vi "Check Start Move.vi"(0 "Bd ID In":T6, 1 "Start All (False)":bool, 2 "Run Mode":enum32{"Sequential", "Parallel"}(ring), 5 "Axis Controls":T1={"Axis 1"={"Axis"=1, "Enable"=FALSE, "Start"=FALSE, "Home"=FALSE, "Stop Type"=0, "Kill"=FALSE}, "Axis 2"={"Axis"=1, "Enable"=FALSE, "Start"=FALSE, "Home"=FALSE, "Stop Type"=0, "Kill"=FALSE}, "Axis 3"={"Axis"=1, "Enable"=FALSE, "Start"=FALSE, "Home"=FALSE, "Stop Type"=0, "Kill"=FALSE}, "Axis 4"={"Axis"=1, "Enable"=FALSE, "Start"=FALSE, "Home"=FALSE, "Stop Type"=0, "Kill"=FALSE}, "Axis 5"={"Axis"=1, "Enable"=FALSE, "Start"=FALSE, "Home"=FALSE, "Stop Type"=0, "Kill"=FALSE}, "Axis 6"={"Axis"=1, "Enable"=FALSE, "Start"=FALSE, "Home"=FALSE, "Stop Type"=0, "Kill"=FALSE}} {"Axis 6"."Stop Type" items=["Decelerate", "Halt", "Kill"]; "Axis 6"."Axis" items=["Axis 1"=1, "Axis 2"=2, "Axis 3"=3, "Axis 4"=4, "Axis 5"=5, "Axis 6"=6, "Axis 7"=7, "Axis 8"=8]; "Axis 5"."Stop Type" items=["Decelerate", "Halt", "Kill"]; "Axis 5"."Axis" items=["Axis 1"=1, "Axis 2"=2, "Axis 3"=3, "Axis 4"=4, "Axis 5"=5, "Axis 6"=6, "Axis 7"=7, "Axis 8"=8]; "Axis 4"."Stop Type" items=["Decelerate", "Halt", "Kill"]; "Axis 4"."Axis" items=["Axis 1"=1, "Axis 2"=2, "Axis 3"=3, "Axis 4"=4, "Axis 5"=5, "Axis 6"=6, "Axis 7"=7, "Axis 8"=8]; "Axis 3"."Stop Type" items=["Decelerate", "Halt", "Kill"]; "Axis 3"."Axis" items=["Axis 1"=1, "Axis 2"=2, "Axis 3"=3, "Axis 4"=4, "Axis 5"=5, "Axis 6"=6, "Axis 7"=7, "Axis 8"=8]; "Axis 2"."Stop Type" items=["Decelerate", "Halt", "Kill"]; "Axis 2"."Axis" items=["Axis 1"=1, "Axis 2"=2, "Axis 3"=3, "Axis 4"=4, "Axis 5"=5, "Axis 6"=6, "Axis 7"=7, "Axis 8"=8]; "Axis 1"."Stop Type" items=["Decelerate", "Halt", "Kill"]; "Axis 1"."Axis" items=["Axis 1"=1, "Axis 2"=2, "Axis 3"=3, "Axis 4"=4, "Axis 5"=5, "Axis 6"=6, "Axis 7"=7, "Axis 8"=8]}, 7 "Units (Encoder Counts)":T5=enum."Degrees", 9 "Stop refnum array":refnum<vi>[](array[refnum]), 11 "error in":errorcluster, 12 "Trajectory Parameters":T4={"Operation Mode (Absolute)"=0, "Blend"=FALSE, "Velocity"=6.0, "Acceleration"=4.0, "Deceleration"=4.0, "Blend Factor"=0, "Permitted Following Error"=1000.0, "S Curve Time"=0} {"Operation Mode (Absolute)" items=["Absolute Position", "Relative Position"]}, 13 "Target Positions":dbl[][](array[numeric])) -> (4 "Bd ID Out":T6, 15 "error out":errorcluster)   [LabVIEW 2010]
doc: "Written specifically for the MultiAxisMove VI. Polls the 'Controls' cluster for a 'Start' or 'Start All' signal. If 'Start All' is true, the singleAxisMultiMove subVI is called for all axes in parallel or sequentially depending on the Run Mode parameter. Otherwise, function checks for a true 'Start' condition on each axes in parallel and calls the singleAxisMultiMove subVI accordingly. \n\nTarget Position is a 2D array where each column is an array of positions for the corresponding axis. That is, the first column is an array of positions for the first axis, the second column is an array of positions for the second axis, etc. etc."
uses:
  Typedefs/Units_Enum.ctl
  Shared/typedefs/Trajectory Parameters.ctl
  Typedefs/AxisSpaceControls_ClusterofAxisControls.ctl
  Typedefs/AxisControls_cluster.ctl
  <vilib>/Motion/FlexMotion/CustomControls/CustomControls.llb/Axis To Control.flx
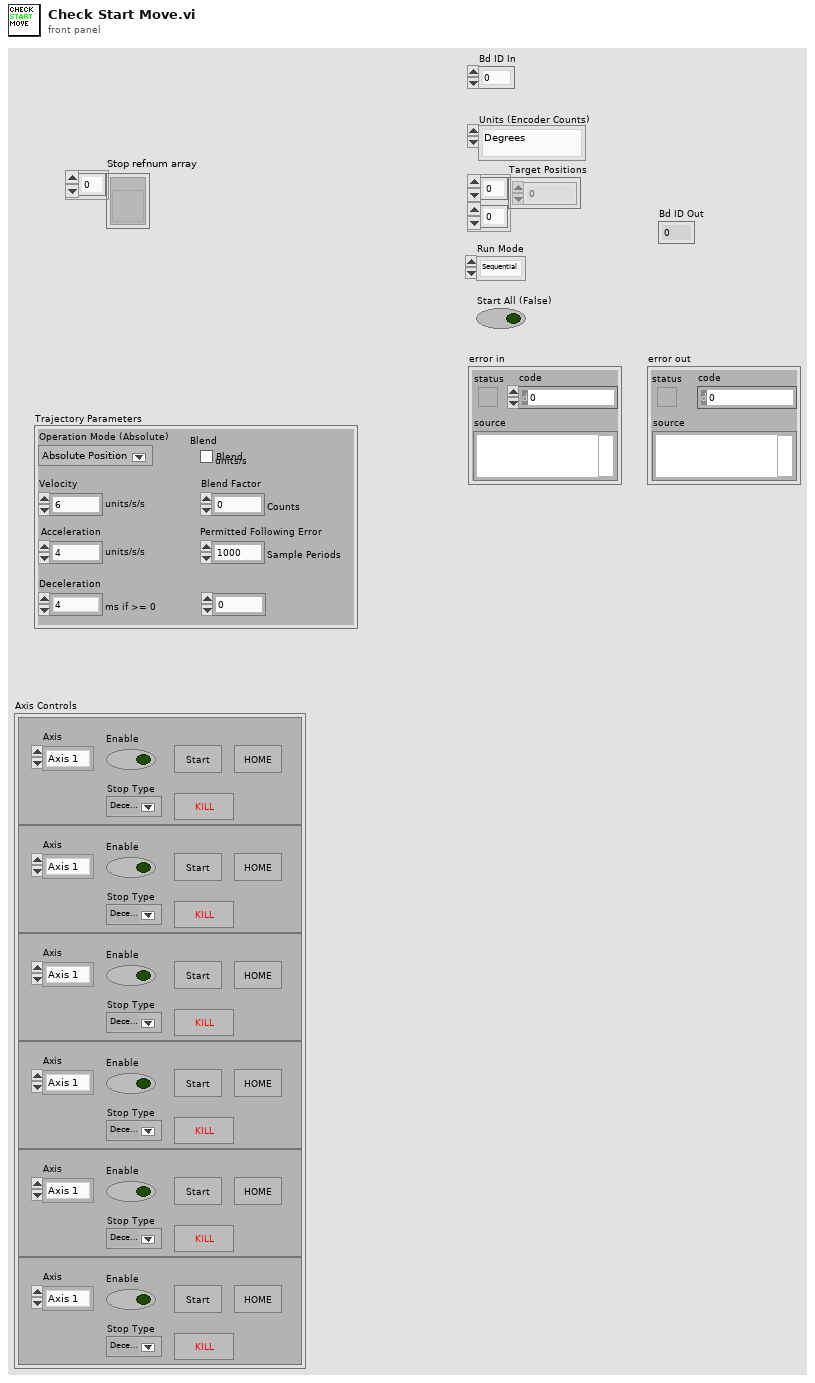
[diagram p1: front panel]
types:
  T1 = typedef "AxisSpaceControls_ClusterofAxisControls.ctl" = cluster{"Axis 1":T2, "Axis 2":T2, "Axis 3":T2, "Axis 4":T2, "Axis 5":T2, "Axis 6":T2}
  T2 = typedef "AxisControls_cluster.ctl" = cluster{"Axis":T3, "Enable":bool, "Start":bool, "Home":bool, "Stop Type":u16, "Kill":bool}
  T3 = typedef "Axis To Control.flx" = u16
  T4 = typedef "Trajectory Parameters.ctl" = cluster{"Operation Mode (Absolute)":u16, "Blend":bool, "Velocity":dbl, "Acceleration":dbl, "Deceleration":dbl, "Blend Factor":i16, "Permitted Following Error":dbl, "S Curve Time":u16}
  T5 = typedef "Units_Enum.ctl" = enum16{"Radians", "Encoder Counts", "Revolutions", "Degrees"}
  T6 = typedef "Bd Id Out" = u8
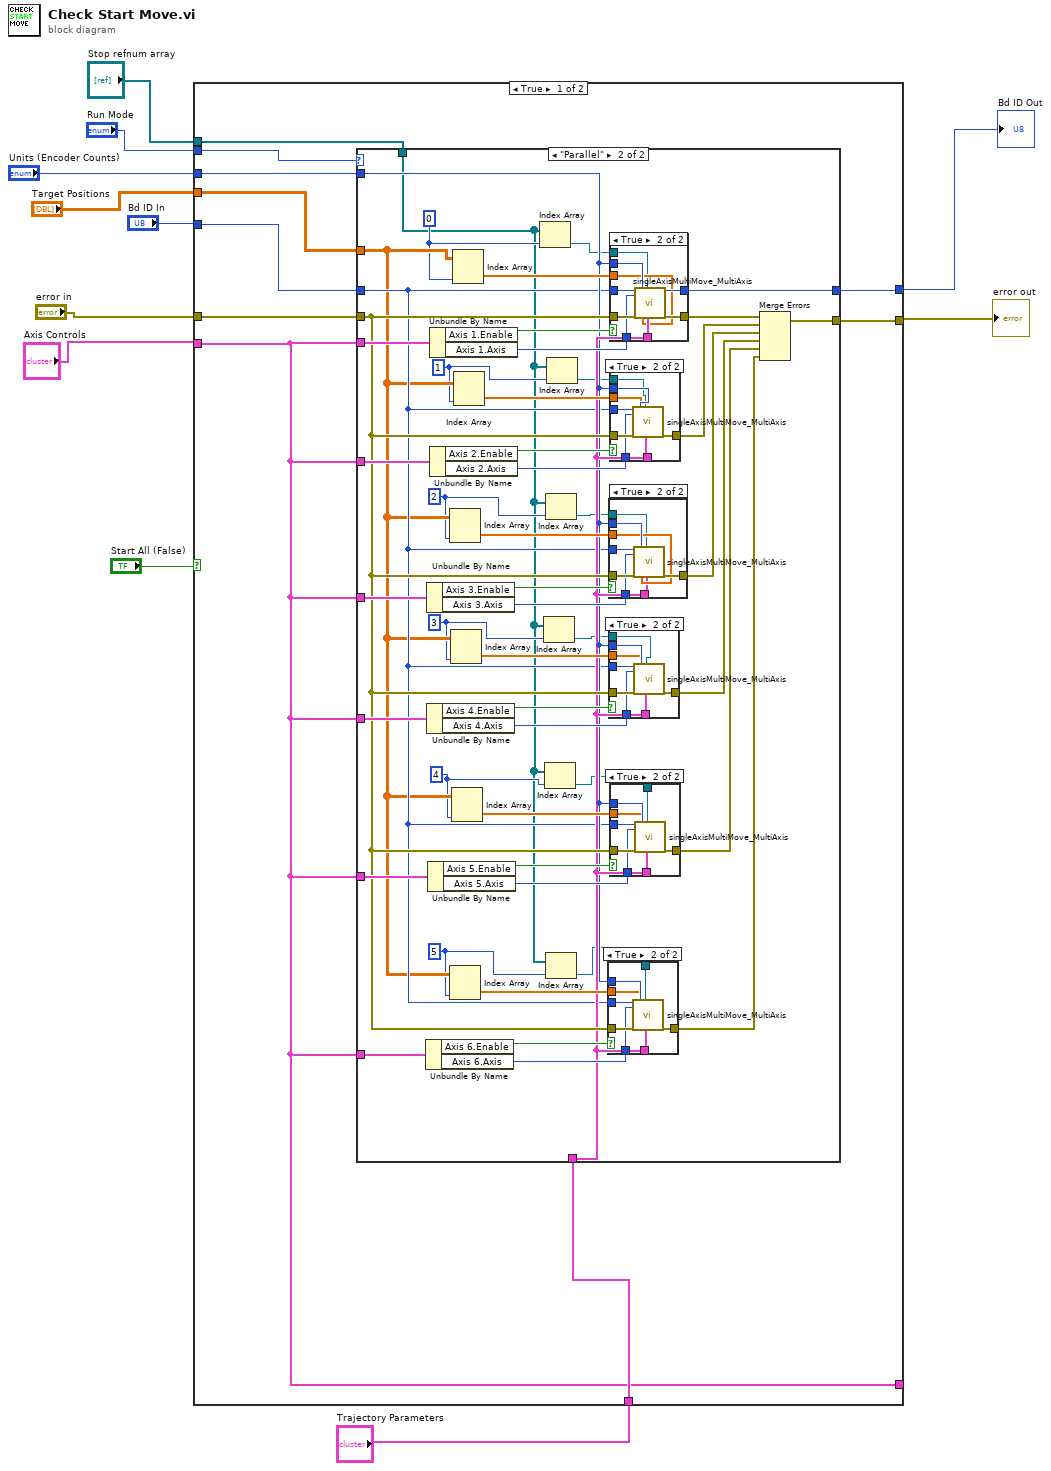
[diagram p0: block diagram]
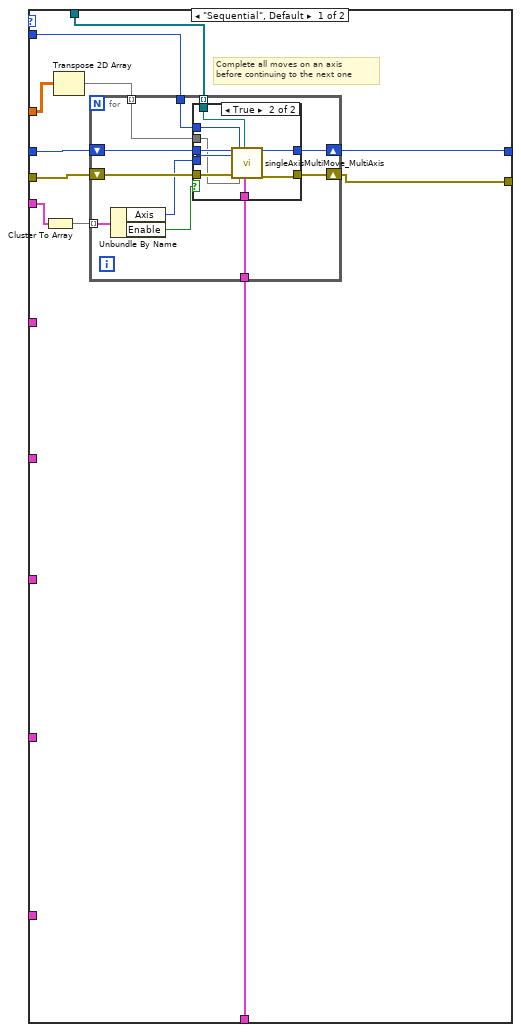
[diagram p2: hidden frame]
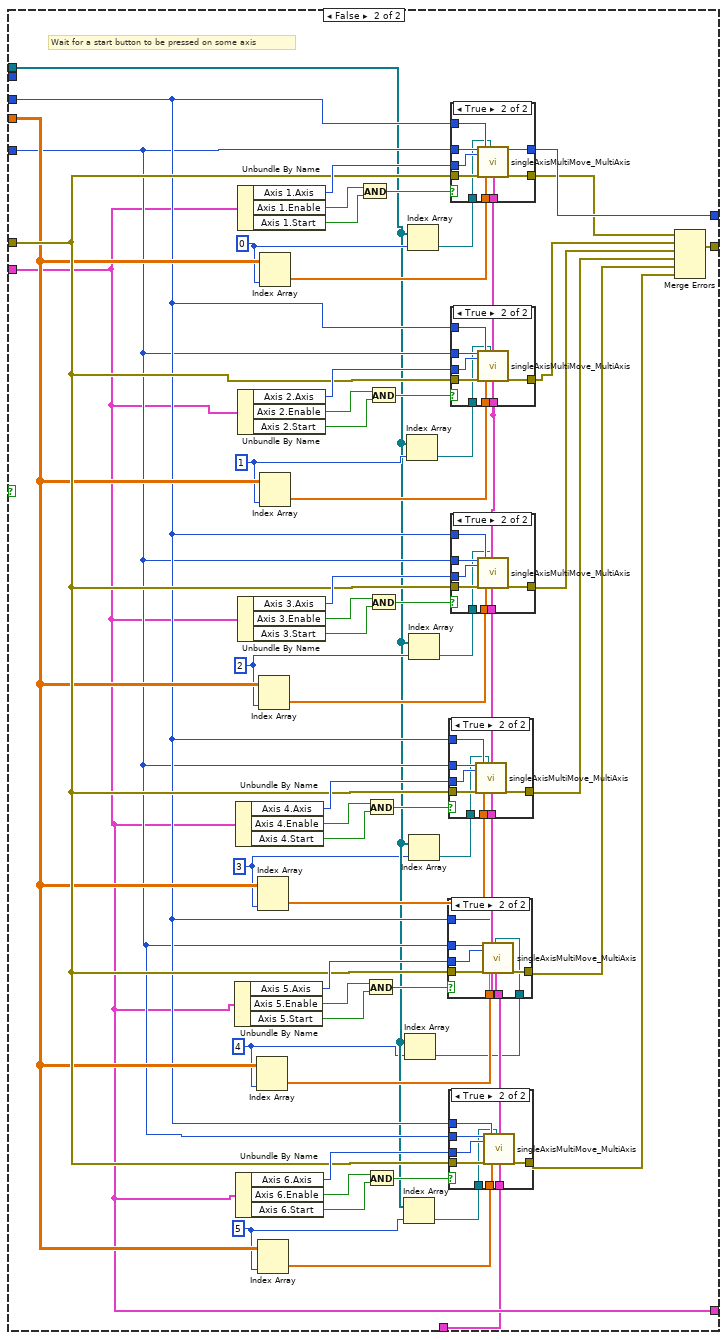
[diagram p10: hidden frame]
diagram:
  n1 = case shown="True" "Start All (False)" {
    tunnel: "Bd ID In" -> [w15 w177]
    tunnel: "error in" -> [w20 w180]
    tunnel: "Target Positions" -> [w17 w179]
    tunnel: "Run Mode" -> [w21 _]
    tunnel: "Axis Controls" -> [w16 w176]
    tunnel: "Trajectory Parameters" -> [w19 w174]
    tunnel: [w18 w216] -> w9
    tunnel: [w16 w176] -> _
    tunnel: [w14 w217] -> w6
    tunnel: "Units (Encoder Counts)" -> [w13 w178]
    tunnel: "Stop refnum array" -> [w12 w167]
    frame True {
      n2 = case shown="\"Parallel\"" w21 {
        tunnel: w20 -> [w32 w73]
        tunnel: w17 -> [w31 w68]
        tunnel: w16 -> [w29 w104]
        tunnel: w15 -> [w28 w70]
        tunnel: w19 -> [w26 w72]
        tunnel: [w25 w102] -> w18
        tunnel: w16 -> [_ w97]
        tunnel: w16 -> [_ w87]
        tunnel: w16 -> [_ w86]
        tunnel: w16 -> [_ w79]
        tunnel: w16 -> [_ w74]
        tunnel: [w24 w83] -> w14
        tunnel: w13 -> [w23 w71]
        tunnel: w12 -> [w22 w56]
        frame "Sequential", Default {
          # "Complete all moves on an axis\nbefore continuing to the next one"
          n3 = Cluster To Array(cluster=w29) -> (array=w27:T2[])
          n4 = Transpose 2D Array(2D array=w31) -> (transposed array=w30:dbl[][])
          n5 = for {
            tunnel: w30 -> [w37] mode=indexing
            tunnel: w27 -> [w41] mode=indexing
            tunnel: w26 -> [w38]
            shift-right: [w36] -> w25
            shift-left: w32 -> [w43]
            tunnel: w23 -> [w35]
            shift-right: [w34] -> w24
            shift-left: w28 -> [w42]
            tunnel: w22 -> [w33] mode=indexing
            n6 = Unbundle By Name(w41) -> ("Axis"=w40:T3, "Enable"=w39:bool)
            n7 = case shown="True" w39 {
              tunnel: w43 -> [w45 w54]
              tunnel: w42 -> [w44 w53]
              tunnel: w40 -> [_ w52]
              tunnel: w38 -> [_ w48]
              tunnel: w37 -> [_ w47]
              tunnel: [w45 w51] -> w36
              tunnel: w35 -> [_ w49]
              tunnel: [w44 w50] -> w34
              tunnel: w33 -> [_ w46]
              frame False {
              }
              frame True {
                n8 = call "singleAxisMultiMove_MultiAxis.vi"("Bd ID"=w53, "Axis"=w52, "error in (no error)"=w54, "Units (Encoder Counts)"=w49, "Target Positions"=w47, "Stop Refnum"=w46, "Trajectory Parameters"=w48) -> ("Bd ID Out"=w50:T6, "error out"=w51:errorcluster)  [unwired: 10 in, 1 out]
              }
            }
          }
        }
        frame "Parallel" {
          w57 = 5 ("disabled index (col)")
          w59 = 4 ("disabled index (col)")
          w61 = 3 ("disabled index (col)")
          w63 = 2 ("disabled index (col)")
          w65 = 1 ("disabled index (col)")
          w66 = 0 ("disabled index (col)")
          n9 = Unbundle By Name(w74) -> ("Axis 6.Enable"=w77:bool, "Axis 6.Axis"=w76:T3)
          n10 = Unbundle By Name(w87) -> ("Axis 3.Enable"=w89:bool, "Axis 3.Axis"=w88:T3)
          n11 = Unbundle By Name(w86) -> ("Axis 4.Enable"=w90:bool, "Axis 4.Axis"=w91:T3)
          n12 = Unbundle By Name(w79) -> ("Axis 5.Enable"=w80:bool, "Axis 5.Axis"=w81:T3)
          n13 = Unbundle By Name(w104) -> ("Axis 1.Enable"=w95:bool, "Axis 1.Axis"=w94:T3)
          n14 = Unbundle By Name(w97) -> ("Axis 2.Enable"=w96:bool, "Axis 2.Axis"=w98:T3)
          n15 = Index Array(array=w68, index (col)=w63) -> (element=w93:dbl[])  [unwired: 1 in]
          n16 = Index Array(array=w68, index (col)=w57) -> (element=w75:dbl[])  [unwired: 1 in]
          n17 = Index Array(array=w68, index (col)=w61) -> (element=w92:dbl[])  [unwired: 1 in]
          n18 = Index Array(array=w68, index (col)=w59) -> (element=w82:dbl[])  [unwired: 1 in]
          n19 = Index Array(array=w68, index (col)=w66) -> (element=w103:dbl[])  [unwired: 1 in]
          n20 = Index Array(array=w68, index (col)=w65) -> (element=w99:dbl[])  [unwired: 1 in]
          n21 = Index Array(array=w56, index=w66) -> (element=w67:refnum<vi>)
          n22 = Index Array(array=w56, index=w61) -> (element=w60:refnum<vi>)
          n23 = Index Array(array=w56, index=w59) -> (element=w58:refnum<vi>)
          n24 = Index Array(array=w56, index=w63) -> (element=w62:refnum<vi>)
          n25 = Index Array(array=w56, index=w57) -> (element=w55:refnum<vi>)
          n26 = Index Array(array=w56, index=w65) -> (element=w64:refnum<vi>)
          n27 = case shown="True" w77 {
            tunnel: w73 -> [w105 w113]
            tunnel: w72 -> [_ w108]
            tunnel: [w105 w112] -> w69
            tunnel: w70 -> [_ w111]
            tunnel: w75 -> [_ w107]
            tunnel: w76 -> [_ w110]
            tunnel: w71 -> [_ w109]
            tunnel: w55 -> [_ w106]
            frame False {
            }
            frame True {
              n28 = call "singleAxisMultiMove_MultiAxis.vi"("Bd ID"=w111, "Axis"=w110, "error in (no error)"=w113, "Units (Encoder Counts)"=w109, "Target Positions"=w107, "Stop Refnum"=w106, "Trajectory Parameters"=w108) -> ("error out"=w112:errorcluster)  [unwired: 10 in, 2 out]
            }
          }
          n29 = case shown="True" w89 {
            tunnel: w73 -> [w132 w140]
            tunnel: w70 -> [_ w139]
            tunnel: w93 -> [_ w135]
            tunnel: w72 -> [_ w134]
            tunnel: [w132 w138] -> w85
            tunnel: w88 -> [_ w137]
            tunnel: w71 -> [_ w136]
            tunnel: w62 -> [_ w133]
            frame False {
            }
            frame True {
              n30 = call "singleAxisMultiMove_MultiAxis.vi"("Bd ID"=w139, "Axis"=w137, "error in (no error)"=w140, "Units (Encoder Counts)"=w136, "Target Positions"=w135, "Stop Refnum"=w133, "Trajectory Parameters"=w134) -> ("error out"=w138:errorcluster)  [unwired: 10 in, 2 out]
            }
          }
          n31 = case shown="True" w90 {
            tunnel: w73 -> [w123 w131]
            tunnel: w72 -> [_ w126]
            tunnel: [w123 w130] -> w84
            tunnel: w70 -> [_ w129]
            tunnel: w92 -> [_ w125]
            tunnel: w91 -> [_ w128]
            tunnel: w71 -> [_ w127]
            tunnel: w60 -> [_ w124]
            frame False {
            }
            frame True {
              n32 = call "singleAxisMultiMove_MultiAxis.vi"("Bd ID"=w129, "Axis"=w128, "error in (no error)"=w131, "Units (Encoder Counts)"=w127, "Target Positions"=w125, "Stop Refnum"=w124, "Trajectory Parameters"=w126) -> ("error out"=w130:errorcluster)  [unwired: 10 in, 2 out]
            }
          }
          n33 = case shown="True" w95 {
            tunnel: w73 -> [w151 w160]
            tunnel: w70 -> [w150 w159]
            tunnel: w103 -> [_ w153]
            tunnel: w72 -> [_ w154]
            tunnel: [w151 w158] -> w100
            tunnel: w94 -> [_ w157]
            tunnel: w71 -> [_ w155]
            tunnel: [w150 w156] -> w83
            tunnel: w67 -> [_ w152]
            frame False {
            }
            frame True {
              n34 = call "singleAxisMultiMove_MultiAxis.vi"("Bd ID"=w159, "Axis"=w157, "error in (no error)"=w160, "Units (Encoder Counts)"=w155, "Target Positions"=w153, "Stop Refnum"=w152, "Trajectory Parameters"=w154) -> ("Bd ID Out"=w156:T6, "error out"=w158:errorcluster)  [unwired: 10 in, 1 out]
            }
          }
          n35 = case shown="True" w96 {
            tunnel: w73 -> [w141 w149]
            tunnel: w72 -> [_ w144]
            tunnel: [w141 w148] -> w101
            tunnel: w70 -> [_ w147]
            tunnel: w99 -> [_ w143]
            tunnel: w98 -> [_ w146]
            tunnel: w71 -> [_ w145]
            tunnel: w64 -> [_ w142]
            frame False {
            }
            frame True {
              n36 = call "singleAxisMultiMove_MultiAxis.vi"("Bd ID"=w147, "Axis"=w146, "error in (no error)"=w149, "Units (Encoder Counts)"=w145, "Target Positions"=w143, "Stop Refnum"=w142, "Trajectory Parameters"=w144) -> ("error out"=w148:errorcluster)  [unwired: 10 in, 2 out]
            }
          }
          n37 = case shown="True" w80 {
            tunnel: w73 -> [w114 w122]
            tunnel: w72 -> [_ w117]
            tunnel: [w114 w121] -> w78
            tunnel: w70 -> [_ w120]
            tunnel: w82 -> [_ w116]
            tunnel: w81 -> [_ w119]
            tunnel: w71 -> [_ w118]
            tunnel: w58 -> [_ w115]
            frame False {
            }
            frame True {
              n38 = call "singleAxisMultiMove_MultiAxis.vi"("Bd ID"=w120, "Axis"=w119, "error in (no error)"=w122, "Units (Encoder Counts)"=w118, "Target Positions"=w116, "Stop Refnum"=w115, "Trajectory Parameters"=w117) -> ("error out"=w121:errorcluster)  [unwired: 10 in, 2 out]
            }
          }
          n39 = Merge Errors(w100, w101, w85, w84, w78, w69) -> (w102:errorcluster)
        }
      }
    }
    frame False {
      w166 = 5 ("disabled index (col)")
      w163 = 4 ("disabled index (col)")
      w162 = 3 ("disabled index (col)")
      w169 = 2 ("disabled index (col)")
      w171 = 1 ("disabled index (col)")
      w172 = 0 ("disabled index (col)")
      # "Wait for a start button to be pressed on some axis"
      n40 = Unbundle By Name(w176) -> ("Axis 5.Axis"=w189:T3, "Axis 5.Enable"=w190:bool, "Axis 5.Start"=w187:bool)
      n41 = Unbundle By Name(w176) -> ("Axis 4.Axis"=w194:T3, "Axis 4.Enable"=w195:bool, "Axis 4.Start"=w192:bool)
      n42 = Unbundle By Name(w176) -> ("Axis 6.Axis"=w184:T3, "Axis 6.Enable"=w185:bool, "Axis 6.Start"=w182:bool)
      n43 = Unbundle By Name(w176) -> ("Axis 1.Axis"=w209:T3, "Axis 1.Enable"=w210:bool, "Axis 1.Start"=w207:bool)
      n44 = Unbundle By Name(w176) -> ("Axis 2.Axis"=w204:T3, "Axis 2.Enable"=w205:bool, "Axis 2.Start"=w202:bool)
      n45 = Unbundle By Name(w176) -> ("Axis 3.Axis"=w199:T3, "Axis 3.Enable"=w200:bool, "Axis 3.Start"=w197:bool)
      n46 = Index Array(array=w179, index (col)=w163) -> (element=w188:dbl[])  [unwired: 1 in]
      n47 = Index Array(array=w179, index (col)=w162) -> (element=w193:dbl[])  [unwired: 1 in]
      n48 = Index Array(array=w179, index (col)=w166) -> (element=w183:dbl[])  [unwired: 1 in]
      n49 = Index Array(array=w179, index (col)=w169) -> (element=w198:dbl[])  [unwired: 1 in]
      n50 = Index Array(array=w179, index (col)=w172) -> (element=w208:dbl[])  [unwired: 1 in]
      n51 = Index Array(array=w179, index (col)=w171) -> (element=w203:dbl[])  [unwired: 1 in]
      n52 = And(x=w210, y=w207) -> (x .and. y?=w211:bool)
      n53 = And(x=w190, y=w187) -> (x .and. y?=w191:bool)
      n54 = And(x=w195, y=w192) -> (x .and. y?=w196:bool)
      n55 = And(x=w185, y=w182) -> (x .and. y?=w186:bool)
      n56 = And(x=w205, y=w202) -> (x .and. y?=w206:bool)
      n57 = And(x=w200, y=w197) -> (x .and. y?=w201:bool)
      n58 = Index Array(array=w167, index=w166) -> (element=w165:refnum<vi>)
      n59 = Index Array(array=w167, index=w163) -> (element=w164:refnum<vi>)
      n60 = Index Array(array=w167, index=w171) -> (element=w170:refnum<vi>)
      n61 = Index Array(array=w167, index=w172) -> (element=w173:refnum<vi>)
      n62 = Index Array(array=w167, index=w169) -> (element=w168:refnum<vi>)
      n63 = Index Array(array=w167, index=w162) -> (element=w161:refnum<vi>)
      n64 = case shown="True" w191 {
        tunnel: w177 -> [_ w235]
        tunnel: [w227 w234] -> w181
        tunnel: w180 -> [w227 w233]
        tunnel: w178 -> [_ w229]
        tunnel: w189 -> [_ w232]
        tunnel: w188 -> [_ w230]
        tunnel: w174 -> [_ w231]
        tunnel: w164 -> [_ w228]
        frame False {
        }
        frame True {
          n65 = call "singleAxisMultiMove_MultiAxis.vi"("Bd ID"=w235, "Axis"=w232, "error in (no error)"=w233, "Units (Encoder Counts)"=w229, "Target Positions"=w230, "Stop Refnum"=w228, "Trajectory Parameters"=w231) -> ("error out"=w234:errorcluster)  [unwired: 10 in, 2 out]
        }
      }
      n66 = case shown="True" w196 {
        tunnel: w177 -> [_ w244]
        tunnel: [w236 w243] -> w212
        tunnel: w180 -> [w236 w242]
        tunnel: w178 -> [_ w240]
        tunnel: w194 -> [_ w241]
        tunnel: w193 -> [_ w239]
        tunnel: w174 -> [_ w238]
        tunnel: w161 -> [_ w237]
        frame False {
        }
        frame True {
          n67 = call "singleAxisMultiMove_MultiAxis.vi"("Bd ID"=w244, "Axis"=w241, "error in (no error)"=w242, "Units (Encoder Counts)"=w240, "Target Positions"=w239, "Stop Refnum"=w237, "Trajectory Parameters"=w238) -> ("error out"=w243:errorcluster)  [unwired: 10 in, 2 out]
        }
      }
      n68 = case shown="True" w186 {
        tunnel: w177 -> [_ w226]
        tunnel: [w218 w225] -> w175
        tunnel: w180 -> [w218 w224]
        tunnel: w178 -> [_ w220]
        tunnel: w184 -> [_ w223]
        tunnel: w183 -> [_ w221]
        tunnel: w174 -> [_ w222]
        tunnel: w165 -> [_ w219]
        frame False {
        }
        frame True {
          n69 = call "singleAxisMultiMove_MultiAxis.vi"("Bd ID"=w226, "Axis"=w223, "error in (no error)"=w224, "Units (Encoder Counts)"=w220, "Target Positions"=w221, "Stop Refnum"=w219, "Trajectory Parameters"=w222) -> ("error out"=w225:errorcluster)  [unwired: 10 in, 2 out]
        }
      }
      n70 = case shown="True" w211 {
        tunnel: [w263 w273] -> w217
        tunnel: w177 -> [w263 w272]
        tunnel: [w264 w271] -> w215
        tunnel: w180 -> [w264 w270]
        tunnel: w178 -> [_ w268]
        tunnel: w209 -> [_ w269]
        tunnel: w208 -> [_ w267]
        tunnel: w174 -> [_ w266]
        tunnel: w173 -> [_ w265]
        frame False {
        }
        frame True {
          n71 = call "singleAxisMultiMove_MultiAxis.vi"("Bd ID"=w272, "Axis"=w269, "error in (no error)"=w270, "Units (Encoder Counts)"=w268, "Target Positions"=w267, "Stop Refnum"=w265, "Trajectory Parameters"=w266) -> ("Bd ID Out"=w273:T6, "error out"=w271:errorcluster)  [unwired: 10 in, 1 out]
        }
      }
      n72 = case shown="True" w206 {
        tunnel: w177 -> [_ w262]
        tunnel: [w254 w261] -> w214
        tunnel: w180 -> [w254 w260]
        tunnel: w178 -> [_ w258]
        tunnel: w204 -> [_ w259]
        tunnel: w203 -> [_ w257]
        tunnel: w174 -> [_ w256]
        tunnel: w170 -> [_ w255]
        frame False {
        }
        frame True {
          n73 = call "singleAxisMultiMove_MultiAxis.vi"("Bd ID"=w262, "Axis"=w259, "error in (no error)"=w260, "Units (Encoder Counts)"=w258, "Target Positions"=w257, "Stop Refnum"=w255, "Trajectory Parameters"=w256) -> ("error out"=w261:errorcluster)  [unwired: 10 in, 2 out]
        }
      }
      n74 = case shown="True" w201 {
        tunnel: w177 -> [_ w253]
        tunnel: [w245 w252] -> w213
        tunnel: w180 -> [w245 w251]
        tunnel: w178 -> [_ w249]
        tunnel: w199 -> [_ w250]
        tunnel: w198 -> [_ w248]
        tunnel: w174 -> [_ w247]
        tunnel: w168 -> [_ w246]
        frame False {
        }
        frame True {
          n75 = call "singleAxisMultiMove_MultiAxis.vi"("Bd ID"=w253, "Axis"=w250, "error in (no error)"=w251, "Units (Encoder Counts)"=w249, "Target Positions"=w248, "Stop Refnum"=w246, "Trajectory Parameters"=w247) -> ("error out"=w252:errorcluster)  [unwired: 10 in, 2 out]
        }
      }
      n76 = Merge Errors(w215, w214, w213, w212, w181, w175) -> (w216:errorcluster)
    }
  }
  "error out" <- w9
  "Bd ID Out" <- w6
